vi "2.- Pruebas con Funciones GPIB.vi"() -> ()   [LabVIEW 2019]
uses:
  Controles/Amp_Frec.ctl
  <vilib>/Utility/error.llb/DialogType.ctl
  QMH_Support/Enqueue Message (Single).vi
  Varios/Globales.vi
  <vilib>/Utility/error.llb/Error Cluster From Error Code.vi
  <vilib>/ErrorRing/Error Ring.xnode
  QMH_Support/Message Queue.lvlib
  QMH_Support/User Event - Stop/User Event - Stop.lvlib
  DS360_GPIB/DS360_GPIB.lvlib
  K2202_GPIB/K2002_GPIB.lvlib
  CNT90_GPIB/CNT90_GPIB.lvlib
panel:
  in  "go_A":bool
  out "CNT90":i32
  out "K2002":i32
  out "DS360":i32
  out "Voltaje a generar":dbl(knob) scale=0.0..10.0
  out "error out":errorcluster
  in  "stop":bool
  in  "generar":bool
  in  "Voltaje a Generar":dbl(slide)=7.0649350649350655 scale=0.0..10.0
  out "voltMon":dbl format="%.2f"
  out "frecMon":dbl format="%.2f"
  # "Ensayo Eléctrico Ponderación A"
  # "Monitoreo"
  # "Frecuencia"
  # "Hz"
  # "Voltaje"
  # "mV"
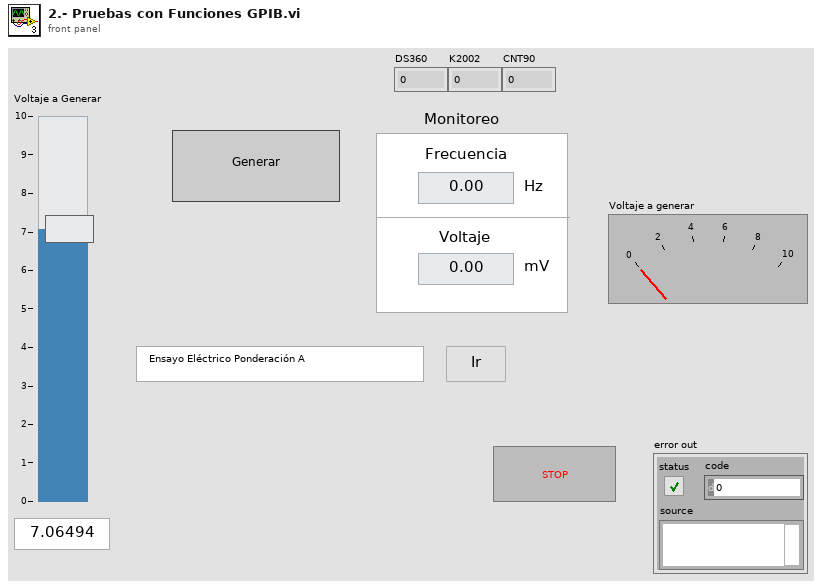
[diagram p1: front panel]
types:
  T1 = typedef "Message Queue.lvlib/All Message Queues.ctl" = cluster{"MHL":refnum<queue>, "DS360":refnum<queue>, "K2002":refnum<queue>, "CNT90":refnum<queue>, "Instrumentos":refnum<queue>}
  T2 = typedef "Amp_Frec.ctl" = cluster{"Ampl":dbl, "Frec":dbl}
  T3 = typedef "DialogType.ctl" = u16
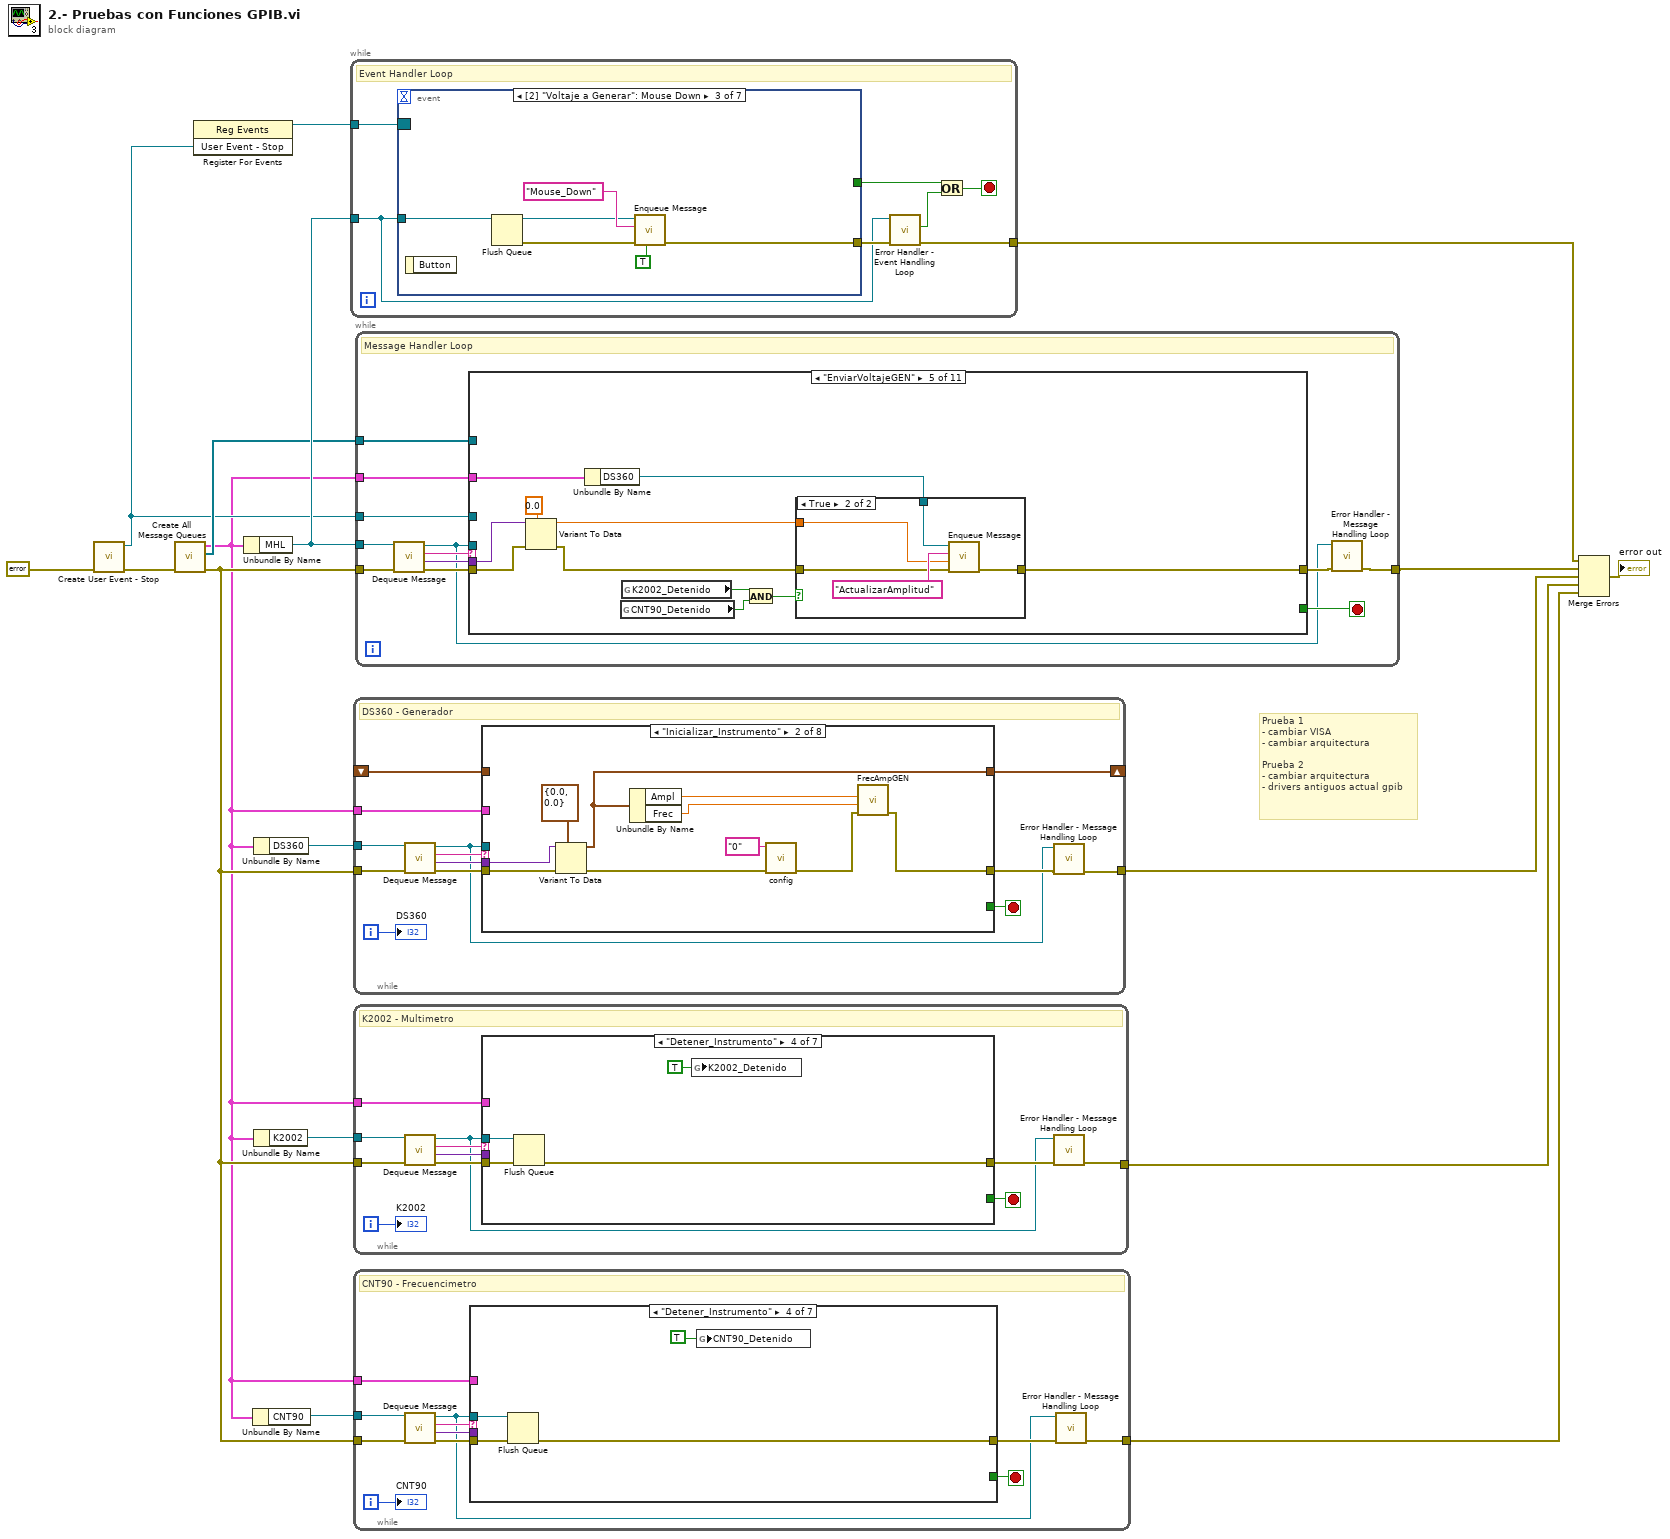
[diagram p0: block diagram]
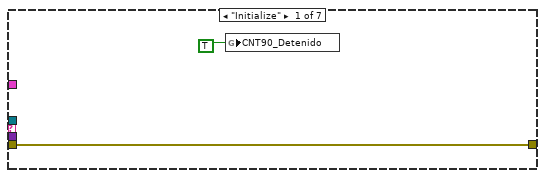
[diagram p2: hidden frame]
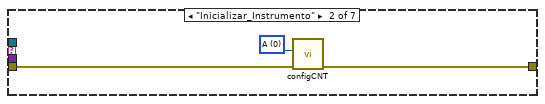
[diagram p3: hidden frame]
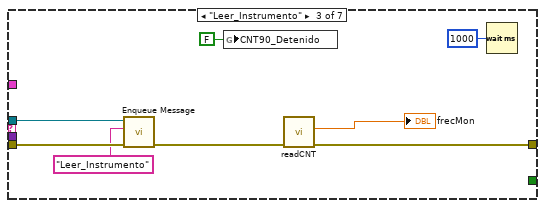
[diagram p4: hidden frame]
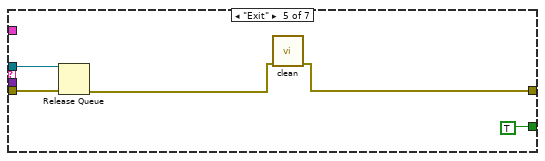
[diagram p5: hidden frame]
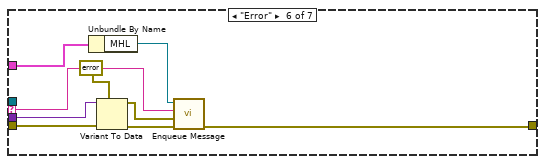
[diagram p6: hidden frame]
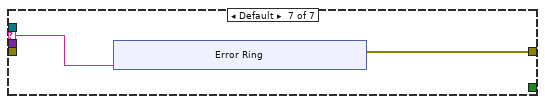
[diagram p7: hidden frame]
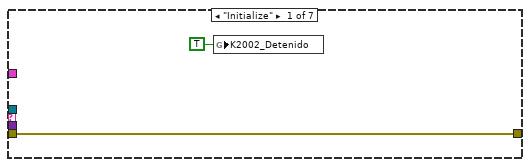
[diagram p8: hidden frame]
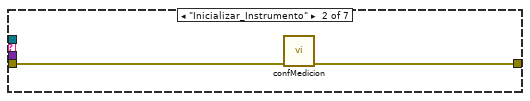
[diagram p9: hidden frame]
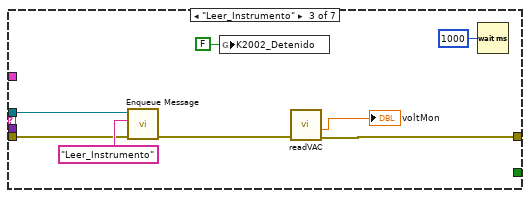
[diagram p10: hidden frame]
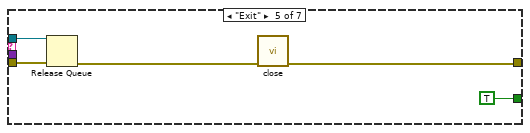
[diagram p11: hidden frame]
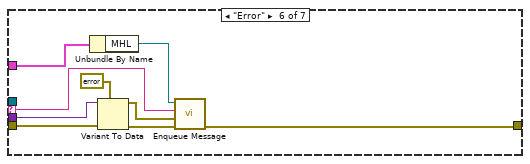
[diagram p12: hidden frame]
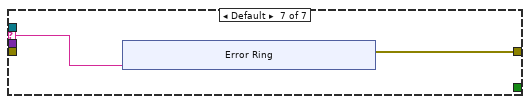
[diagram p13: hidden frame]
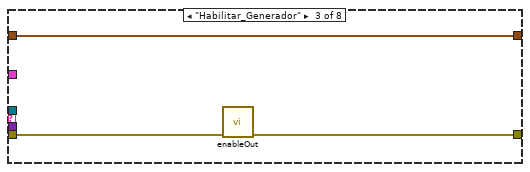
[diagram p15: hidden frame]
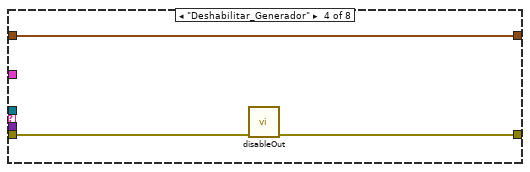
[diagram p16: hidden frame]
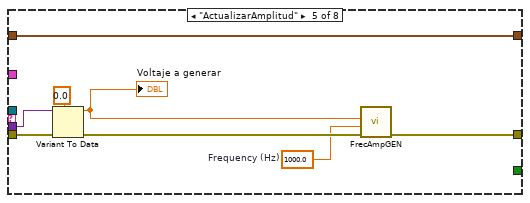
[diagram p17: hidden frame]
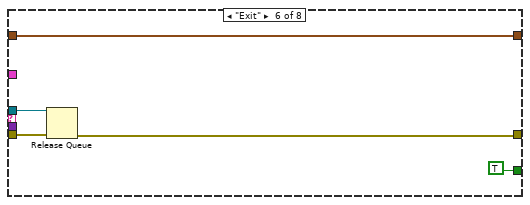
[diagram p18: hidden frame]
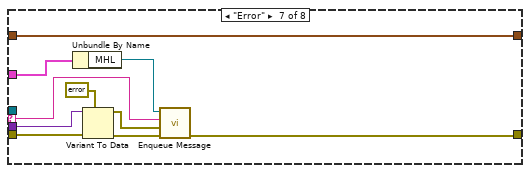
[diagram p19: hidden frame]
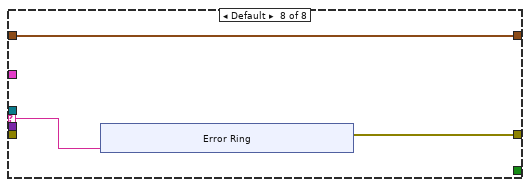
[diagram p20: hidden frame]
diagram:
  # "Prueba 1\n- cambiar VISA\n- cambiar arquitectura\n\nPrueba 2\n- cambiar arquitectura\n- drivers antiguos actual gpib"
  n1 = call "Create User Event - Stop.vi"("error in (no error)"=errorcluster {"status"=FALSE, "code"=0, "source"=""}) -> ("error out"=w9:errorcluster, "User Event - Stop"=w8:refnum<user-event>)  [unwired: 9 in]
  n2 = call "Create All Message Queues.vi"("error in (no error)"=w9) -> ("error out"=w6:errorcluster, "Queues Array"=w11:refnum<queue>[], "Message Queues out"=w3:T1)  [unwired: 8 in]
  n3 = register-events(w8) -> (reference out=w7:refnum<event-registration>)  [unwired: 2 in, 1 out]
  n4 = Unbundle By Name(w3) -> ("MHL"=w17:refnum<queue>)
  n5 = Unbundle By Name(w3) -> ("CNT90"=w4:refnum<queue>)
  n6 = Unbundle By Name(w3) -> ("DS360"=w16:refnum<queue>)
  n7 = Unbundle By Name(w3) -> ("K2002"=w5:refnum<queue>)
  n8 = while {
    tunnel: w17 -> [w21]
    tunnel: [w22] -> w15
    tunnel: w7 -> [w24]
    stop <- w18 stop-if-true
    # "Event Handler Loop"
    n9 = event shown="[2] \"Voltaje a Generar\": Mouse Down" {
      selector: w24 -> [_ _ _ _ _ _ _]
      dyn-events: _ -> [_ _ _ _ _ _ _]
      timeout: _ -> [_ _ _ _ _ _ _]
      tunnel: w21 -> [w26 w29 w38 w46 w51 w59 _]
      tunnel: [w25 w28 w39 w45 w52 w57 _] -> w23
      tunnel: [_ _ _ _ _ _ TRUE] -> w20
      event "go_A": Value Change {
        n10 = event-data() -> ()  [unwired: 1 in, 1 out]
        n11 = call-poly "Enqueue Message.vi"("Message"="Inicializar_Instrumento_A" ("message"), "Message Queue"=w26) -> ("error out"=w25:errorcluster)  [unwired: 8 in, 1 out]
      }
      event "generar": Value Change {
        n12 = event-data() -> ("NewVal"=w30:bool)  [unwired: 1 in]
        n13 = Flush Queue(queue=w29) -> (queue out=w31:refnum<queue>, error out=w32:errorcluster)  [unwired: 1 in, 1 out]
        n14 = Select(t="iniciarGEN_A1" ("message"), s=w30, f="detenerGEN" ("message")) -> (s? t:f=w35:string)
        n15 = call-poly "Enqueue Message.vi"("Priority Message? (F)"=TRUE, "error in (no error)"=w32, "Message Data"="A1" ("message"), "Message"=w35, "Message Queue"=w31) -> ("error out"=w28:errorcluster)  [unwired: 5 in, 1 out]
      }
      event "Voltaje a Generar": Mouse Down {
        n16 = event-data() -> ()  [unwired: 1 in, 1 out]
        n17 = Flush Queue(queue=w38) -> (queue out=w40:refnum<queue>, error out=w41:errorcluster)  [unwired: 1 in, 1 out]
        n18 = call-poly "Enqueue Message.vi"("Priority Message? (F)"=TRUE, "error in (no error)"=w41, "Message"="Mouse_Down" ("message"), "Message Queue"=w40) -> ("error out"=w39:errorcluster)  [unwired: 6 in, 1 out]
      }
      event "Voltaje a Generar": Value Change {
        n19 = event-data() -> ("NewVal"=w44:dbl)  [unwired: 1 in]
        n20 = Flush Queue(queue=w46) -> (queue out=w47:refnum<queue>, error out=w48:errorcluster)  [unwired: 1 in, 1 out]
        n21 = call-poly "Enqueue Message.vi"("Priority Message? (F)"=TRUE, "error in (no error)"=w48, "Message Data"=w44, "Message"="EnviarVoltajeGEN" ("message"), "Message Queue"=w47) -> ("error out"=w45:errorcluster)  [unwired: 5 in, 1 out]
      }
      event "Voltaje a Generar": Mouse Up {
        n22 = event-data() -> ()  [unwired: 1 in, 1 out]
        n23 = Flush Queue(queue=w51) -> (queue out=w53:refnum<queue>, error out=w54:errorcluster)  [unwired: 1 in, 1 out]
        n24 = call-poly "Enqueue Message.vi"("Priority Message? (F)"=TRUE, "error in (no error)"=w54, "Message"="Reiniciar_Lectura" ("message"), "Message Queue"=w53) -> ("error out"=w52:errorcluster)  [unwired: 6 in, 1 out]
      }
      event "stop": Value Change {
        n25 = event-data() -> ()  [unwired: 1 in, 1 out]
        n26 = call-poly "Enqueue Message.vi"("Message"="Exit", "Message Queue"=w59) -> ("error out"=w57:errorcluster)  [unwired: 8 in, 1 out]
      }
      event User Event {
        n27 = event-data() -> ()  [unwired: 1 in, 1 out]
      }
    }
    n28 = call "Error Handler - Event Handling Loop.vi"("error in (no error)"=w23, "Message Queue"=w21) -> ("dup error in"=w22:errorcluster, "Error?"=w19:bool)  [unwired: 7 in, 1 out]
    n29 = Or(x=w20, y=w19) -> (x .or. y?=w18:bool)
  }
  n30 = while {
    tunnel: w16 -> [w73]
    tunnel: w6 -> [w72]
    tunnel: [w62] -> w13
    tunnel: w3 -> [w68]
    shift-right: [w65] -> _
    shift-left: _ -> [w64]
    i -> [w66]
    stop <- w67 stop-if-true
    # "DS360 - Generador"
    n31 = call "Dequeue Message.vi"("error in (no error)"=w72, "Message Queue"=w73) -> ("error out"=w71:errorcluster, "Message Data"=w69:variant, "Message"=w70:string, "dup Message Queue"=w61:refnum<queue>)  [unwired: 6 in]
    n32 = case shown="\"Inicializar_Instrumento\"" w70 {
      selector: w70 -> [_ _ _ _ _ _ w107 w117]
      tunnel: w71 -> [w74 w85 w87 w90 w98 w104 w110 _]
      tunnel: w69 -> [_ w83 _ _ w97 _ w109 _]
      tunnel: w61 -> [_ _ _ _ _ w103 _ _]
      tunnel: [w74 w78 w86 w89 w94 w100 w106 w116] -> w63
      tunnel: w68 -> [_ _ _ _ _ _ w108 _]
      tunnel: [_ _ _ _ _ TRUE _ _] -> w67
      tunnel: [w75 w82 w88 w91 w96 w101 w105 w115] -> w65
      tunnel: w64 -> [w75 _ w88 w91 w96 w101 w105 w115]
      frame "Initialize" {
      }
      frame "Inicializar_Instrumento" {
        n33 = Variant To Data(error in=w85, type=T2 {"Ampl"=0.0, "Frec"=0.0}, Variant=w83) -> (data=w82:T2, error out=w81:errorcluster)
        n34 = Unbundle By Name(w82) -> ("Ampl"=w77:dbl, "Frec"=w76:dbl)
        n35 = call "config.vi"("error in (no error)"=w81, "Impedancia"="0") -> ("error out"=w79:errorcluster)  [unwired: 9 in]
        n36 = call "FrecAmpGEN.vi"("error in (no error)"=w79, "Frec (Hz)"=w76, "Amplitud (Vrms)"=w77) -> ("error out"=w78:errorcluster)  [unwired: 8 in]
      }
      frame "Habilitar_Generador" {
        n37 = call "enableOut.vi"("error in (no error)"=w87) -> ("error out"=w86:errorcluster)  [unwired: 10 in]
      }
      frame "Deshabilitar_Generador" {
        n38 = call "disableOut.vi"("error in (no error)"=w90) -> ("error out"=w89:errorcluster)  [unwired: 10 in]
      }
      frame "ActualizarAmplitud" {
        w92 = 1000.0  # Frequency (Hz)
        n39 = Variant To Data(error in=w98, type=0.0, Variant=w97) -> (data=w93:dbl, error out=w95:errorcluster)
        "Voltaje a generar" <- w93
        n40 = call "FrecAmpGEN.vi"("error in (no error)"=w95, "Frec (Hz)"=w92, "Amplitud (Vrms)"=w93) -> ("error out"=w94:errorcluster)  [unwired: 8 in]
      }
      frame "Exit" {
        n41 = Release Queue(queue=w103, error in (no error)=w104) -> (error out=w100:errorcluster)  [unwired: 1 in, 2 out]
      }
      frame "Error" {
        n42 = Unbundle By Name(w108) -> ("MHL"=w111:refnum<queue>)
        n43 = Variant To Data(error in=w110, type=errorcluster {"status"=FALSE, "code"=0, "source"=""} ("error constant"), Variant=w109) -> (data=w112:errorcluster, error out=w113:errorcluster)
        n44 = call-poly "Enqueue Message.vi"("error in (no error)"=w113, "Message Data"=w112, "Message"=w107, "Message Queue"=w111) -> ("error out"=w106:errorcluster)  [unwired: 6 in, 1 out]
      }
      frame Default {
        n45 = xnode "Error Ring"("parameter 0"=w117) -> ("error out"=w116:errorcluster)
      }
    }
    n46 = call "Error Handler - Message Handling Loop.vi"("error in (no error)"=w63, "Message Queue"=w61) -> ("dup error in"=w62:errorcluster)  [unwired: 8 in, 1 out]
    "DS360" <- w66
  }
  n47 = while {
    tunnel: w5 -> [w135]
    tunnel: w6 -> [w134]
    tunnel: w3 -> [w130]
    tunnel: [w126] -> w2
    i -> [w128]
    stop <- w129 stop-if-true
    # "K2002 - Multimetro"
    n48 = call "Dequeue Message.vi"("error in (no error)"=w134, "Message Queue"=w135) -> ("error out"=w133:errorcluster, "Message Data"=w131:variant, "Message"=w132:string, "dup Message Queue"=w125:refnum<queue>)  [unwired: 6 in]
    n49 = case shown="\"Detener_Instrumento\"" w132 {
      selector: w132 -> [_ _ _ _ _ w158 w167]
      tunnel: w133 -> [w136 w139 w145 w151 w156 w161 _]
      tunnel: w131 -> [_ _ _ _ _ w160 _]
      tunnel: w125 -> [_ _ w144 w149 w155 _ _]
      tunnel: [w136 w138 w141 w150 w152 w157 w166] -> w127
      tunnel: w130 -> [_ _ _ _ _ w159 _]
      tunnel: [_ _ _ _ TRUE _ _] -> w129
      frame "Initialize" {
        n50 = global write "Globales.vi" "K2002_Detenido"(TRUE ("K2002_Detenido")) -> ()
      }
      frame "Inicializar_Instrumento" {
        n51 = call "confMedicion.vi"("error in (no error)"=w139) -> ("error out"=w138:errorcluster)  [unwired: 10 in]
      }
      frame "Leer_Instrumento" {
        n52 = call-poly "Enqueue Message.vi"("error in (no error)"=w145, "Message"="Leer_Instrumento", "Message Queue"=w144) -> ("error out"=w142:errorcluster)  [unwired: 7 in, 1 out]
        n53 = global write "Globales.vi" "K2002_Detenido"(FALSE ("K2002_Detenido")) -> ()
        n54 = call "readVAC.vi"("error in (no error)"=w142) -> ("error out"=w141:errorcluster, "medicion"=→"voltMon":dbl)  [unwired: 8 in, 1 out]
        n55 = Wait (ms)(milliseconds to wait=u32 1000) -> ()  [unwired: 1 out]
      }
      frame "Detener_Instrumento" {
        n56 = Flush Queue(queue=w149, error in (no error)=w151) -> (error out=w150:errorcluster)  [unwired: 2 out]
        n57 = global write "Globales.vi" "K2002_Detenido"(TRUE ("K2002_Detenido")) -> ()
      }
      frame "Exit" {
        n58 = Release Queue(queue=w155, error in (no error)=w156) -> (error out=w153:errorcluster)  [unwired: 1 in, 2 out]
        n59 = call "close.vi"("error in (no error)"=w153) -> ("error out"=w152:errorcluster)  [unwired: 10 in]
      }
      frame "Error" {
        n60 = Unbundle By Name(w159) -> ("MHL"=w162:refnum<queue>)
        n61 = Variant To Data(error in=w161, type=errorcluster {"status"=FALSE, "code"=0, "source"=""} ("error constant"), Variant=w160) -> (data=w163:errorcluster, error out=w164:errorcluster)
        n62 = call-poly "Enqueue Message.vi"("error in (no error)"=w164, "Message Data"=w163, "Message"=w158, "Message Queue"=w162) -> ("error out"=w157:errorcluster)  [unwired: 6 in, 1 out]
      }
      frame Default {
        n63 = xnode "Error Ring"("parameter 0"=w167) -> ("error out"=w166:errorcluster)
      }
    }
    n64 = call "Error Handler - Message Handling Loop.vi"("error in (no error)"=w127, "Message Queue"=w125) -> ("dup error in"=w126:errorcluster)  [unwired: 8 in, 1 out]
    "K2002" <- w128
  }
  n65 = while {
    tunnel: w4 -> [w185]
    tunnel: w6 -> [w184]
    tunnel: w3 -> [w180]
    tunnel: [w176] -> w1
    i -> [w178]
    stop <- w179 stop-if-true
    # "CNT90 - Frecuencimetro"
    n66 = call "Dequeue Message.vi"("error in (no error)"=w184, "Message Queue"=w185) -> ("error out"=w183:errorcluster, "Message Data"=w181:variant, "Message"=w182:string, "dup Message Queue"=w175:refnum<queue>)  [unwired: 6 in]
    n67 = case shown="\"Detener_Instrumento\"" w182 {
      selector: w182 -> [_ _ _ _ _ w209 w218]
      tunnel: w183 -> [w187 w190 w198 w202 w207 w212 _]
      tunnel: w181 -> [_ _ _ _ _ w211 _]
      tunnel: w175 -> [_ _ w194 w200 w206 _ _]
      tunnel: [w187 w189 w197 w201 w203 w208 w217] -> w177
      tunnel: w180 -> [_ _ _ _ _ w210 _]
      tunnel: [_ _ _ _ TRUE _ _] -> w179
      frame "Initialize" {
        n68 = global write "Globales.vi" "CNT90_Detenido"(TRUE ("CNT90_Detenido")) -> ()
      }
      frame "Inicializar_Instrumento" {
        w188 = 0 items=["A", "B"] ("Channel  1")
        n69 = call "configCNT.vi"("error in (no error)"=w190, "Channel  1"=w188) -> ("error out"=w189:errorcluster)  [unwired: 9 in]
      }
      frame "Leer_Instrumento" {
        n70 = call-poly "Enqueue Message.vi"("error in (no error)"=w198, "Message"="Leer_Instrumento", "Message Queue"=w194) -> ("error out"=w195:errorcluster)  [unwired: 7 in, 1 out]
        n71 = global write "Globales.vi" "CNT90_Detenido"(FALSE ("CNT90_Detenido")) -> ()
        n72 = call "readCNT.vi"("error in (no error)"=w195) -> ("error out"=w197:errorcluster, "medicion"=→"frecMon":dbl)  [unwired: 9 in]
        n73 = Wait (ms)(milliseconds to wait=u32 1000) -> ()  [unwired: 1 out]
      }
      frame "Detener_Instrumento" {
        n74 = Flush Queue(queue=w200, error in (no error)=w202) -> (error out=w201:errorcluster)  [unwired: 2 out]
        n75 = global write "Globales.vi" "CNT90_Detenido"(TRUE ("CNT90_Detenido")) -> ()
      }
      frame "Exit" {
        n76 = Release Queue(queue=w206, error in (no error)=w207) -> (error out=w204:errorcluster)  [unwired: 1 in, 2 out]
        n77 = call "clean.vi"("error in (no error)"=w204) -> ("error out"=w203:errorcluster)  [unwired: 10 in]
      }
      frame "Error" {
        n78 = Unbundle By Name(w210) -> ("MHL"=w213:refnum<queue>)
        n79 = Variant To Data(error in=w212, type=errorcluster {"status"=FALSE, "code"=0, "source"=""} ("error constant"), Variant=w211) -> (data=w214:errorcluster, error out=w215:errorcluster)
        n80 = call-poly "Enqueue Message.vi"("error in (no error)"=w215, "Message Data"=w214, "Message"=w209, "Message Queue"=w213) -> ("error out"=w208:errorcluster)  [unwired: 6 in, 1 out]
      }
      frame Default {
        n81 = xnode "Error Ring"("parameter 0"=w218) -> ("error out"=w217:errorcluster)
      }
    }
    n82 = call "Error Handler - Message Handling Loop.vi"("error in (no error)"=w177, "Message Queue"=w175) -> ("dup error in"=w176:errorcluster)  [unwired: 8 in, 1 out]
    "CNT90" <- w178
  }
  n83 = while {
    tunnel: w17 -> [w237]
    tunnel: w6 -> [w236]
    tunnel: [w228] -> w14
    tunnel: w11 -> [w232]
    tunnel: w8 -> [w230]
    tunnel: w3 -> [w226]
    stop <- w231 stop-if-true
    # "Message Handler Loop"
    n84 = call "Dequeue Message.vi"("error in (no error)"=w236, "Message Queue"=w237) -> ("error out"=w233:errorcluster, "Message Data"=w234:variant, "Message"=w235:string, "dup Message Queue"=w227:refnum<queue>)  [unwired: 6 in]
    n85 = case shown="\"EnviarVoltajeGEN\"" w235 {
      selector: w235 -> [_ _ _ _ _ _ _ _ w320 _ w335]
      tunnel: w234 -> [_ _ _ _ w279 _ w303 _ _ w325 _]
      tunnel: w233 -> [w239 w251 w262 w267 w280 w294 w304 w312 w317 w328 _]
      tunnel: w227 -> [_ _ _ _ _ _ _ _ _ w326 _]
      tunnel: [w238 w249 w253 w263 w274 w288 w298 w310 w316 w327 w334] -> w229
      tunnel: w232 -> [_ _ _ _ _ _ _ _ w321 _ _]
      tunnel: [_ _ _ _ _ _ _ _ TRUE _ _] -> w231
      tunnel: w230 -> [_ _ _ _ _ _ _ _ w315 _ _]
      tunnel: w226 -> [_ w247 w261 w266 w278 w293 w302 w311 _ _ _]
      frame "Initialize" {
        n86 = invoke class="VI" method="Default Vals.Reinit All"(error in=w239) -> (error out=w238:errorcluster)  [unwired: 2 in, 2 out]
      }
      frame "Inicializar_Instrumento_A" {
        w248 = "Inicializar_Instrumento" ("Message")
        n87 = Unbundle By Name(w247) -> ("CNT90"=w244:refnum<queue>, "K2002"=w245:refnum<queue>, "DS360"=w246:refnum<queue>)
        n88 = local read "Voltaje a Generar"() -> (w241:dbl)
        n89 = Bundle By Name(cluster=T2 {"Ampl"=0.0, "Frec"=0.0}, "Ampl"=w241, "Frec"=1000.0) -> (w242:T2)
        n90 = call-poly "Enqueue Message.vi"("error in (no error)"=w251, "Message Data"=w242, "Message"=w248, "Message Queue"=w246) -> ("error out"=w252:errorcluster)  [unwired: 6 in, 1 out]
        n91 = call-poly "Enqueue Message.vi"("error in (no error)"=w252, "Message"=w248, "Message Queue"=w245) -> ("error out"=w250:errorcluster)  [unwired: 7 in, 1 out]
        n92 = call-poly "Enqueue Message.vi"("error in (no error)"=w250, "Message"=w248, "Message Queue"=w244) -> ("error out"=w249:errorcluster)  [unwired: 7 in, 1 out]
      }
      frame "iniciarGEN_A1" {
        w256 = "Leer_Instrumento" ("Message")
        n93 = Unbundle By Name(w261) -> ("CNT90"=w257:refnum<queue>, "K2002"=w258:refnum<queue>, "DS360"=w260:refnum<queue>)
        n94 = call-poly "Enqueue Message.vi"("error in (no error)"=w262, "Message"="Habilitar_Generador", "Message Queue"=w260) -> ("error out"=w255:errorcluster)  [unwired: 7 in, 1 out]
        n95 = call-poly "Enqueue Message.vi"("error in (no error)"=w255, "Message"=w256, "Message Queue"=w258) -> ("error out"=w254:errorcluster)  [unwired: 7 in, 1 out]
        n96 = call-poly "Enqueue Message.vi"("error in (no error)"=w254, "Message"=w256, "Message Queue"=w257) -> ("error out"=w253:errorcluster)  [unwired: 7 in, 1 out]
      }
      frame "Mouse_Down" {
        w268 = TRUE ("Priority Message? (F)")
        w269 = "Detener_Instrumento" ("Message")
        n97 = Unbundle By Name(w266) -> ("CNT90"=w264:refnum<queue>, "K2002"=w265:refnum<queue>)
        n98 = call-poly "Enqueue Message.vi"("Priority Message? (F)"=w268, "error in (no error)"=w267, "Message"=w269, "Message Queue"=w265) -> ("error out"=w270:errorcluster)  [unwired: 6 in, 1 out]
        n99 = call-poly "Enqueue Message.vi"("Priority Message? (F)"=w268, "error in (no error)"=w270, "Message"=w269, "Message Queue"=w264) -> ("error out"=w263:errorcluster)  [unwired: 6 in, 1 out]
      }
      frame "EnviarVoltajeGEN" {
        n100 = Variant To Data(error in=w280, type=0.0, Variant=w279) -> (data=w275:dbl, error out=w276:errorcluster)
        n101 = Unbundle By Name(w278) -> ("DS360"=w277:refnum<queue>)
        n102 = global read "Globales.vi" "CNT90_Detenido"() -> (w272:bool)
        n103 = global read "Globales.vi" "K2002_Detenido"() -> (w273:bool)
        n104 = And(x=w273, y=w272) -> (x .and. y?=w271:bool)
        n105 = case shown="True" w271 {
          tunnel: w277 -> [_ w286]
          tunnel: w276 -> [w282 w285]
          tunnel: w275 -> [_ w284]
          tunnel: [w282 w283] -> w274
          frame False {
          }
          frame True {
            n106 = call-poly "Enqueue Message.vi"("error in (no error)"=w285, "Message Data"=w284, "Message"="ActualizarAmplitud", "Message Queue"=w286) -> ("error out"=w283:errorcluster)  [unwired: 6 in, 1 out]
          }
        }
      }
      frame "Reiniciar_Lectura" {
        w290 = "Leer_Instrumento" ("Message")
        n107 = Unbundle By Name(w293) -> ("CNT90"=w291:refnum<queue>, "K2002"=w292:refnum<queue>)
        n108 = call-poly "Enqueue Message.vi"("error in (no error)"=w294, "Message"=w290, "Message Queue"=w292) -> ("error out"=w289:errorcluster)  [unwired: 7 in, 1 out]
        n109 = call-poly "Enqueue Message.vi"("error in (no error)"=w289, "Message"=w290, "Message Queue"=w291) -> ("error out"=w288:errorcluster)  [unwired: 7 in, 1 out]
      }
      frame "Leer_Instrumento" {
        w297 = TRUE ("Priority Message? (F)")
        w299 = "Leer_Instrumento" ("Message")
        n110 = Variant To Data(error in=w304, type=0.0, Variant=w303) -> (error out=w301:errorcluster)  [unwired: 1 out]
        n111 = Unbundle By Name(w302) -> ("K2002"=w296:refnum<queue>, "CNT90"=w295:refnum<queue>)  [unwired: 1 out]
        n112 = call-poly "Enqueue Message.vi"("Priority Message? (F)"=w297, "error in (no error)"=w301, "Message"=w299, "Message Queue"=w295) -> ("error out"=w300:errorcluster)  [unwired: 6 in, 1 out]
        n113 = call-poly "Enqueue Message.vi"("Priority Message? (F)"=w297, "error in (no error)"=w300, "Message"=w299, "Message Queue"=w296) -> ("error out"=w298:errorcluster)  [unwired: 6 in, 1 out]
      }
      frame "detenerGEN" {
        w306 = "Detener_Instruemento" ("Message")
        w309 = 0.0 ("frecMon")
        n114 = Unbundle By Name(w311) -> ("CNT90"=w307:refnum<queue>, "K2002"=w308:refnum<queue>, "DS360"=w314:refnum<queue>)
        n115 = call-poly "Enqueue Message.vi"("error in (no error)"=w312, "Message"="Deshabilitar_Generador", "Message Queue"=w314) -> ("error out"=w310:errorcluster)  [unwired: 7 in, 1 out]
        n116 = call-poly "Enqueue Message.vi"("Message"=w306, "Message Queue"=w308) -> ()  [unwired: 8 in, 2 out]
        n117 = call-poly "Enqueue Message.vi"("Message"=w306, "Message Queue"=w307) -> ()  [unwired: 8 in, 2 out]
        n118 = local write "frecMon"(w309) -> ()
        n119 = local write "voltMon"(w309) -> ()
      }
      frame "Exit" {
        n120 = for {
          tunnel: w321 -> [w324] mode=indexing
          tunnel: w320 -> [w323]
          tunnel: TRUE -> [w322]
          n121 = call-poly "Enqueue Message.vi"("Priority Message? (F)"=w322, "Message"=w323, "Message Queue"=w324) -> ()  [unwired: 7 in, 2 out]
        }
        n122 = call "Fire User Event - Stop.vi"("error in (no error)"=w317, "User Event - Stop"=w315) -> ("error out"=w316:errorcluster)  [unwired: 9 in]
      }
      frame "Error" {
        w332 = T3 1 items=["no dialog", "OK message", "continue or stop message", "OK message + warnings", "continue/stop + warnings"] ("type of dialog (OK msg:1)")
        n123 = Variant To Data(error in=w328, type=errorcluster {"status"=FALSE, "code"=0, "source"=""} ("error out"), Variant=w325) -> (data=w330:errorcluster, error out=w329:errorcluster)
        n124 = call <vilib>:"Simple Error Handler.vi"("type of dialog (OK msg:1)"=w332, "error in (no error)"=w330) -> ()  [unwired: 3 in, 5 out]
        n125 = call-poly "Enqueue Message.vi"("error in (no error)"=w329, "Message"="Exit", "Message Queue"=w326) -> ("error out"=w327:errorcluster)  [unwired: 7 in, 1 out]
      }
      frame Default {
        n126 = xnode "Error Ring"("parameter 0"=w335) -> ("error out"=w334:errorcluster)
      }
    }
    n127 = call "Error Handler - Message Handling Loop.vi"("error in (no error)"=w229, "Message Queue"=w227) -> ("dup error in"=w228:errorcluster)  [unwired: 8 in, 1 out]
  }
  n128 = Merge Errors(w15, w14, w13, w2, w1) -> (→"error out":errorcluster)
